vi "ChParamSetRef.vi"(4 "Init":bool, 5 "Number Of Retry in":refnum<vi>, 6 "Retry Delay in":refnum<vi>, 7 "Current Threshold in":refnum<vi>, 8 "Current Threshold [A] in":refnum<vi>) -> (0 "Number Of Retry out":refnum<vi>, 1 "Retry Delay Set out":refnum<vi>, 2 "Channel On Delay out":refnum<vi>)   [LabVIEW 2010]
panel:
  out "Current Threshold [A] in 2":refnum<vi>
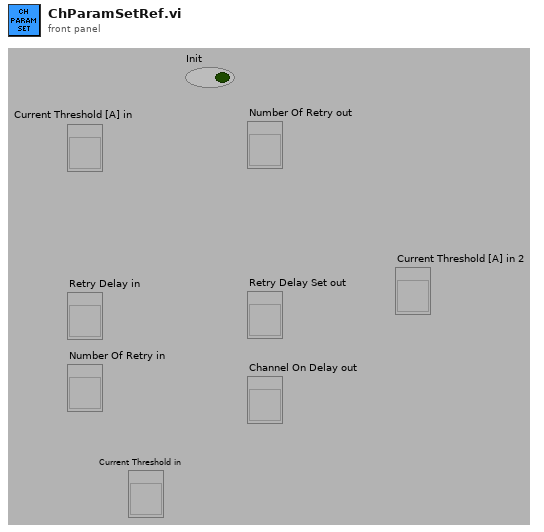
[diagram p1: front panel]
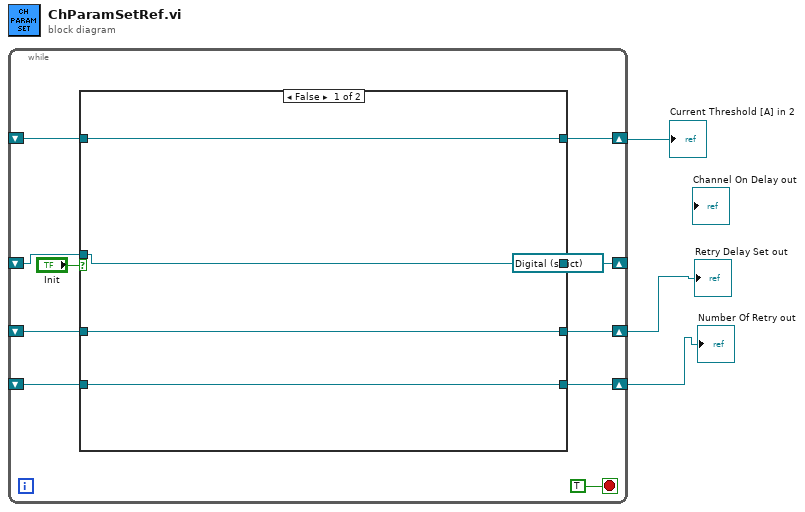
[diagram p0: block diagram]
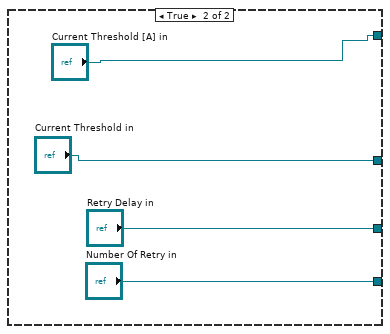
[diagram p2: hidden frame]
diagram:
  n1 = while {
    shift-right: [w12] -> w1
    shift-left: _ -> [w8]
    shift-right: [w11] -> _
    shift-left: _ -> [w7]
    shift-right: [w10] -> w3
    shift-left: _ -> [w6]
    shift-right: [w9] -> w2
    shift-left: _ -> [w5]
    stop <- TRUE stop-if-true
    (unwired) refnum<vi> refnum ("Current Threshold in")
    n2 = case shown="False" "Init" {
      tunnel: [w17 "Current Threshold [A] in"] -> w12
      tunnel: [w16 "Current Threshold in"] -> w11
      tunnel: [w15 "Retry Delay in"] -> w10
      tunnel: [w14 "Number Of Retry in"] -> w9
      tunnel: w8 -> [w17 _]
      tunnel: w7 -> [w16 _]
      tunnel: w6 -> [w15 _]
      tunnel: w5 -> [w14 _]
      frame False {
      }
      frame True {
      }
    }
  }
  "Retry Delay Set out" <- w3
  "Number Of Retry out" <- w2
  "Current Threshold [A] in 2" <- w1
